vi "rotg - Givens Rotation Parameters.vi"   [LabVIEW 2020, in "NI_AALBLAS.lvlib"]
doc: "Creates the parameters used in the rot - Givens Rotation VI."
uses:
  <vilib>/Analysis/NI_AALBLAS.lvlib
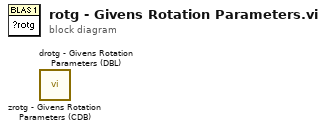
[diagram p0: block diagram]
diagram:
  n1 = call <vilib>:"zrotg - Givens Rotation Parameters (CDB).vi"() -> ()  [unwired: 7 in, 5 out]
  n2 = call <vilib>:"drotg - Givens Rotation Parameters (DBL).vi"() -> ()  [unwired: 7 in, 5 out]
